vi "Habersine(SubVI).vi"(11 "아이템 이름":string[][](array[string])) -> (3 "distance[m]":dbl)   [LabVIEW 2023]
panel:
  out "x-y 2":dbl
  out "x-y":dbl
  out "lon2":dbl
  out "lon1":dbl
  out "lat2":dbl
  out "lat1":dbl
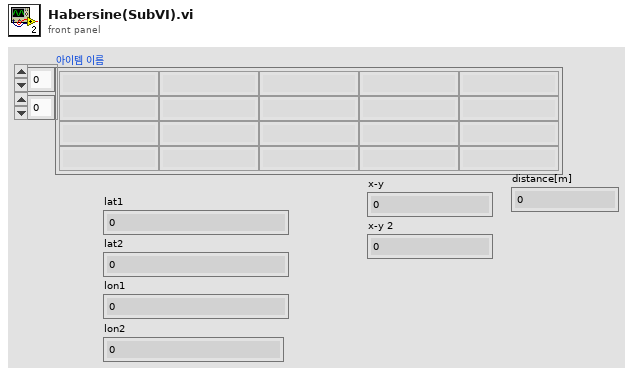
[diagram p1: front panel]
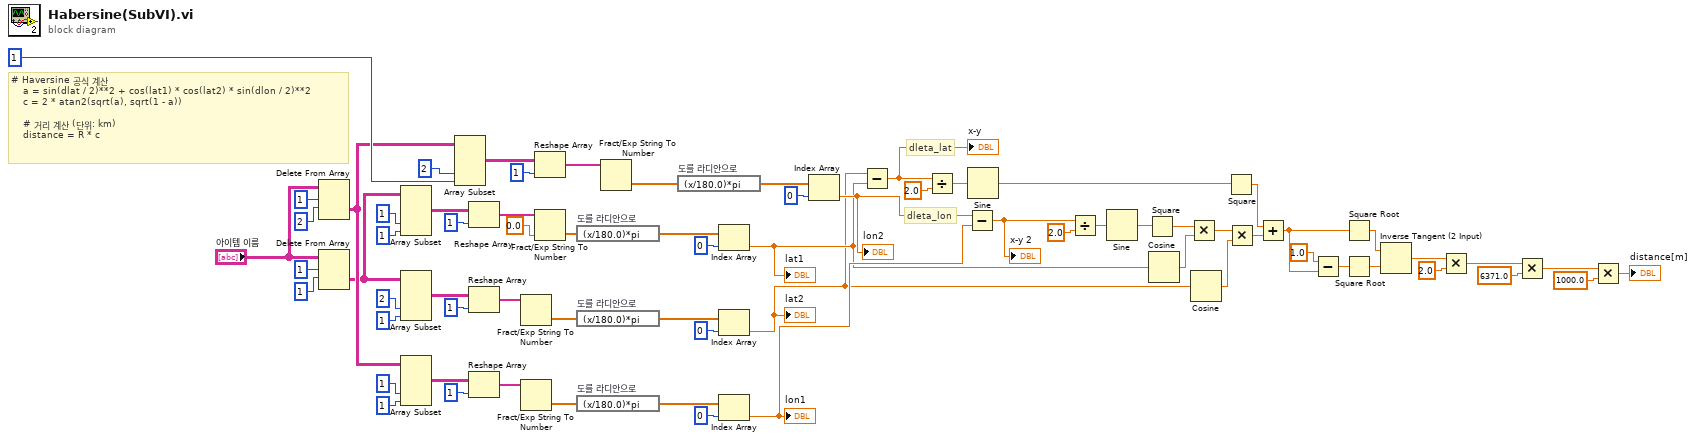
[diagram p0: block diagram]
diagram:
  # "dleta_lon"
  # "dleta_lat"
  # "# Haversine 공식 계산\n    a = sin(dlat / 2)**2 + cos(lat1) * cos(lat2) * sin(dlon / 2)**2\n    c = 2 * atan2(sqrt(a), sqrt(1 - a))\n\n    # 거리 계산 (단위: km)\n    distance = R * c"
  n1 = Delete From Array(array="아이템 이름", length=1 ("길이"), index (row)=2 ("인덱스 (행)")) -> (deleted portion=w62:string[][])  [unwired: 1 in, 1 out]
  n2 = Delete From Array(array="아이템 이름", length=1 ("길이"), index (row)=1 ("인덱스 (행)")) -> (deleted portion=w49:string[][])  [unwired: 1 in, 1 out]
  n3 = Array Subset(array=w49, index (col)=1 ("인덱스"), length (col)=1 ("길이")) -> (w52:string[][])  [unwired: 2 in]
  n4 = Array Subset(array=w49, index (col)=2 ("인덱스"), length (col)=1 ("길이")) -> (w50:string[][])  [unwired: 2 in]
  n5 = Array Subset(array=w62, index (col)=1 ("인덱스"), length (col)=1 ("길이")) -> (w59:string[][])  [unwired: 2 in]
  n6 = Array Subset(array=w62, index (col)=2 ("인덱스"), length (col)=1 ("길이")) -> (w61:string[][])  [unwired: 2 in]
  n7 = Reshape Array(w52, 1 ("차원 크기")) -> (w54:string[])
  n8 = Reshape Array(w50, 1 ("차원 크기")) -> (w55:string[])
  n9 = Reshape Array(w59, 1 ("차원 크기")) -> (w57:string[])
  n10 = Fract/Exp String To Number(string=w55) -> (number=w42:dbl[])  [unwired: 3 in, 1 out]
  n11 = Fract/Exp String To Number(string=w57) -> (number=w41:dbl[])  [unwired: 3 in, 1 out]
  n12 = Reshape Array(w61, 1 ("차원 크기")) -> (w56:string[])
  n13 = Fract/Exp String To Number(string=w54, default (0 dbl)=0.0 ("기본(0 DBL)")) -> (number=w39:dbl[])  [unwired: 2 in, 1 out]
  n14 = expression code="(x/180.0)*pi" "도를 라디안으로"(w39) -> (w38:dbl[])
  n15 = expression code="(x/180.0)*pi" "도를 라디안으로"(w42) -> (w35:dbl[])
  n16 = expression code="(x/180.0)*pi" "도를 라디안으로"(w41) -> (w33:dbl[])
  n17 = Fract/Exp String To Number(string=w56) -> (number=w40:dbl[])  [unwired: 3 in, 1 out]
  n18 = expression code="(x/180.0)*pi" "도를 라디안으로"(w40) -> (w31:dbl[])
  n19 = Index Array(array=w38, index=0 ("인덱스")) -> (element=w5:dbl)
  "lat1" <- w5
  n20 = Index Array(array=w35, index=0 ("인덱스")) -> (element=w4:dbl)
  "lat2" <- w4
  n21 = Index Array(array=w33, index=0 ("인덱스")) -> (element=w6:dbl)
  "lon1" <- w6
  n22 = Index Array(array=w31, index=0 ("인덱스")) -> (element=w7:dbl)
  "lon2" <- w7
  n23 = Subtract(x=w4, y=w5) -> (x-y=w30:dbl)
  "x-y" <- w30
  n24 = Divide(x=w30, y=2.0) -> (x/y=w28:dbl)
  n25 = Subtract(x=w7, y=w6) -> (x-y=w23:dbl)
  "x-y 2" <- w23
  n26 = Sine(x=w28) -> (sin(x)=w27:dbl)
  n27 = Divide(x=w23, y=2.0) -> (x/y=w25:dbl)
  n28 = Sine(x=w25) -> (sin(x)=w26:dbl)
  n29 = Square(x=w26) -> (x^2=w22:dbl)
  n30 = Cosine(x=w5) -> (cos(x)=w21:dbl)
  n31 = Multiply(x=w22, y=w21) -> (x*y=w20:dbl)
  n32 = Cosine(x=w4) -> (cos(x)=w19:dbl)
  n33 = Square(x=w27) -> (x^2=w11:dbl)
  n34 = Multiply(x=w20, y=w19) -> (x*y=w12:dbl)
  n35 = Add(x=w11, y=w12) -> (x+y=w10:dbl)
  n36 = Subtract(x=1.0, y=w10) -> (x-y=w17:dbl)
  n37 = Square Root(x=w10) -> (sqrt(x)=w9:dbl)
  n38 = Square Root(x=w17) -> (sqrt(x)=w8:dbl)
  n39 = Inverse Tangent (2 Input)(1:w8, 2:w9) -> (0:w15:dbl)
  n40 = Multiply(x=w15, y=2.0) -> (x*y=w13:dbl)
  n41 = Multiply(x=w13, y=6371.0) -> (x*y=w3:dbl)
  n42 = Multiply(x=w3, y=1000.0) -> (x*y=→"distance[m]":dbl)
